vi "Main.vi"(11 "Module Admin":refnum<class "Delacor_lib_QMH_Module Admin.lvclass">) -> ()   [LabVIEW 2024, in "Logger.lvlib"]
doc: "This template is based off of the Queued Message Handler design pattern and the Queued Message Handler project template that ships with LabVIEW.\n\nThe main difference is that the queue is private to this module and communication between modules is performed via Broadcast and Request events.\n\nRequest events are wrapped in public API methods and are handled in the Event Handling Loop (EHL) of this VI. Any module can register for Broadcast events sent by this module. The EHL generates messages based on user interface actions.\n\nThe Message Handling Loop (MHL) processes messages generated by the EHL, or by other messages. The messages are string values, so new messages can be added easily to the Message Cases case structure in the MHL. Each message cluster can also provide an optional value for Message Data, which is a variant that can be converted to whatever message-specific data is required.\n_____\nBased on DQMH Project Template 7.0.0.1280."
uses:
  Logger.lvlib
  <vilib>/Delacor/Delacor QMH/Libraries/Module Admin_class/Delacor_lib_QMH_Module Admin.lvclass
  Module Data--cluster.ctl
  <vilib>/Delacor/Delacor QMH/Libraries/Message Queue_class/Delacor_lib_QMH_Message Queue.lvclass/Delacor_lib_QMH_Message Queue.ctl
  Stop Argument--cluster.ctl
  <vilib>/Delacor/Delacor QMH/Libraries/Module Admin_class/Delacor_lib_QMH_Module Admin.lvclass/Delacor_lib_QMH_Module Admin.ctl
  <vilib>/Utility/miscctls.llb/LVPointTypeDef.ctl
  <vilib>/Delacor/Delacor QMH/Libraries/Message Queue_class/Delacor_lib_QMH_Enqueue Message (Single).vi
  <vilib>/Delacor/Delacor QMH/Libraries/Module Admin_class/Delacor_lib_QMH_Get External Launch.vi
  <vilib>/Delacor/Delacor QMH/Libraries/Message Queue_class/Delacor_lib_QMH_Message Queue.lvclass
panel:
  out "error out":errorcluster
  out "Status":string
  in  "Simulate MHL Error":bool
  in  "Simulate EHL Error":bool
  # "This template is for the DQMH framework. See the block diagram for more information on how to use this template."
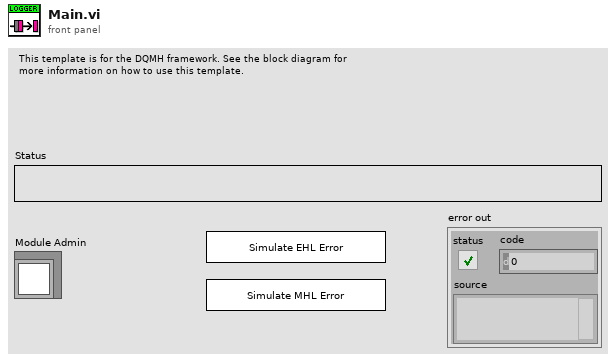
[diagram p1: front panel]
types:
  T1 = typedef "Logger.lvlib/Request Events--cluster.ctl" = cluster{"Stop Module":refnum<user-event>, "Show Panel":refnum<user-event>, "Hide Panel":refnum<user-event>, "Get Module Execution Status":refnum<user-event>, "Show Diagram":refnum<user-event>}
  T2 = typedef "Logger.lvlib/Module Data--cluster.ctl" = cluster{"Status":string}
  T3 = enum32{"invalid lock state", "Not Locked", "Locked (No Password)", "Password-protected"}
  T4 = typedef "Logger.lvlib/Stop Argument--cluster.ctl" = cluster{"Origin":string, "Exit via Stop Module Req?":bool, "Wait for Module to stop?":bool}
  T5 = typedef "LVPointTypeDef.ctl" = cluster{"Horizontal":i16, "Vertical":i16}
  T6 = enum32{"Invalid", "Standard", "Closed", "Hidden", "Minimized", "Maximized"}
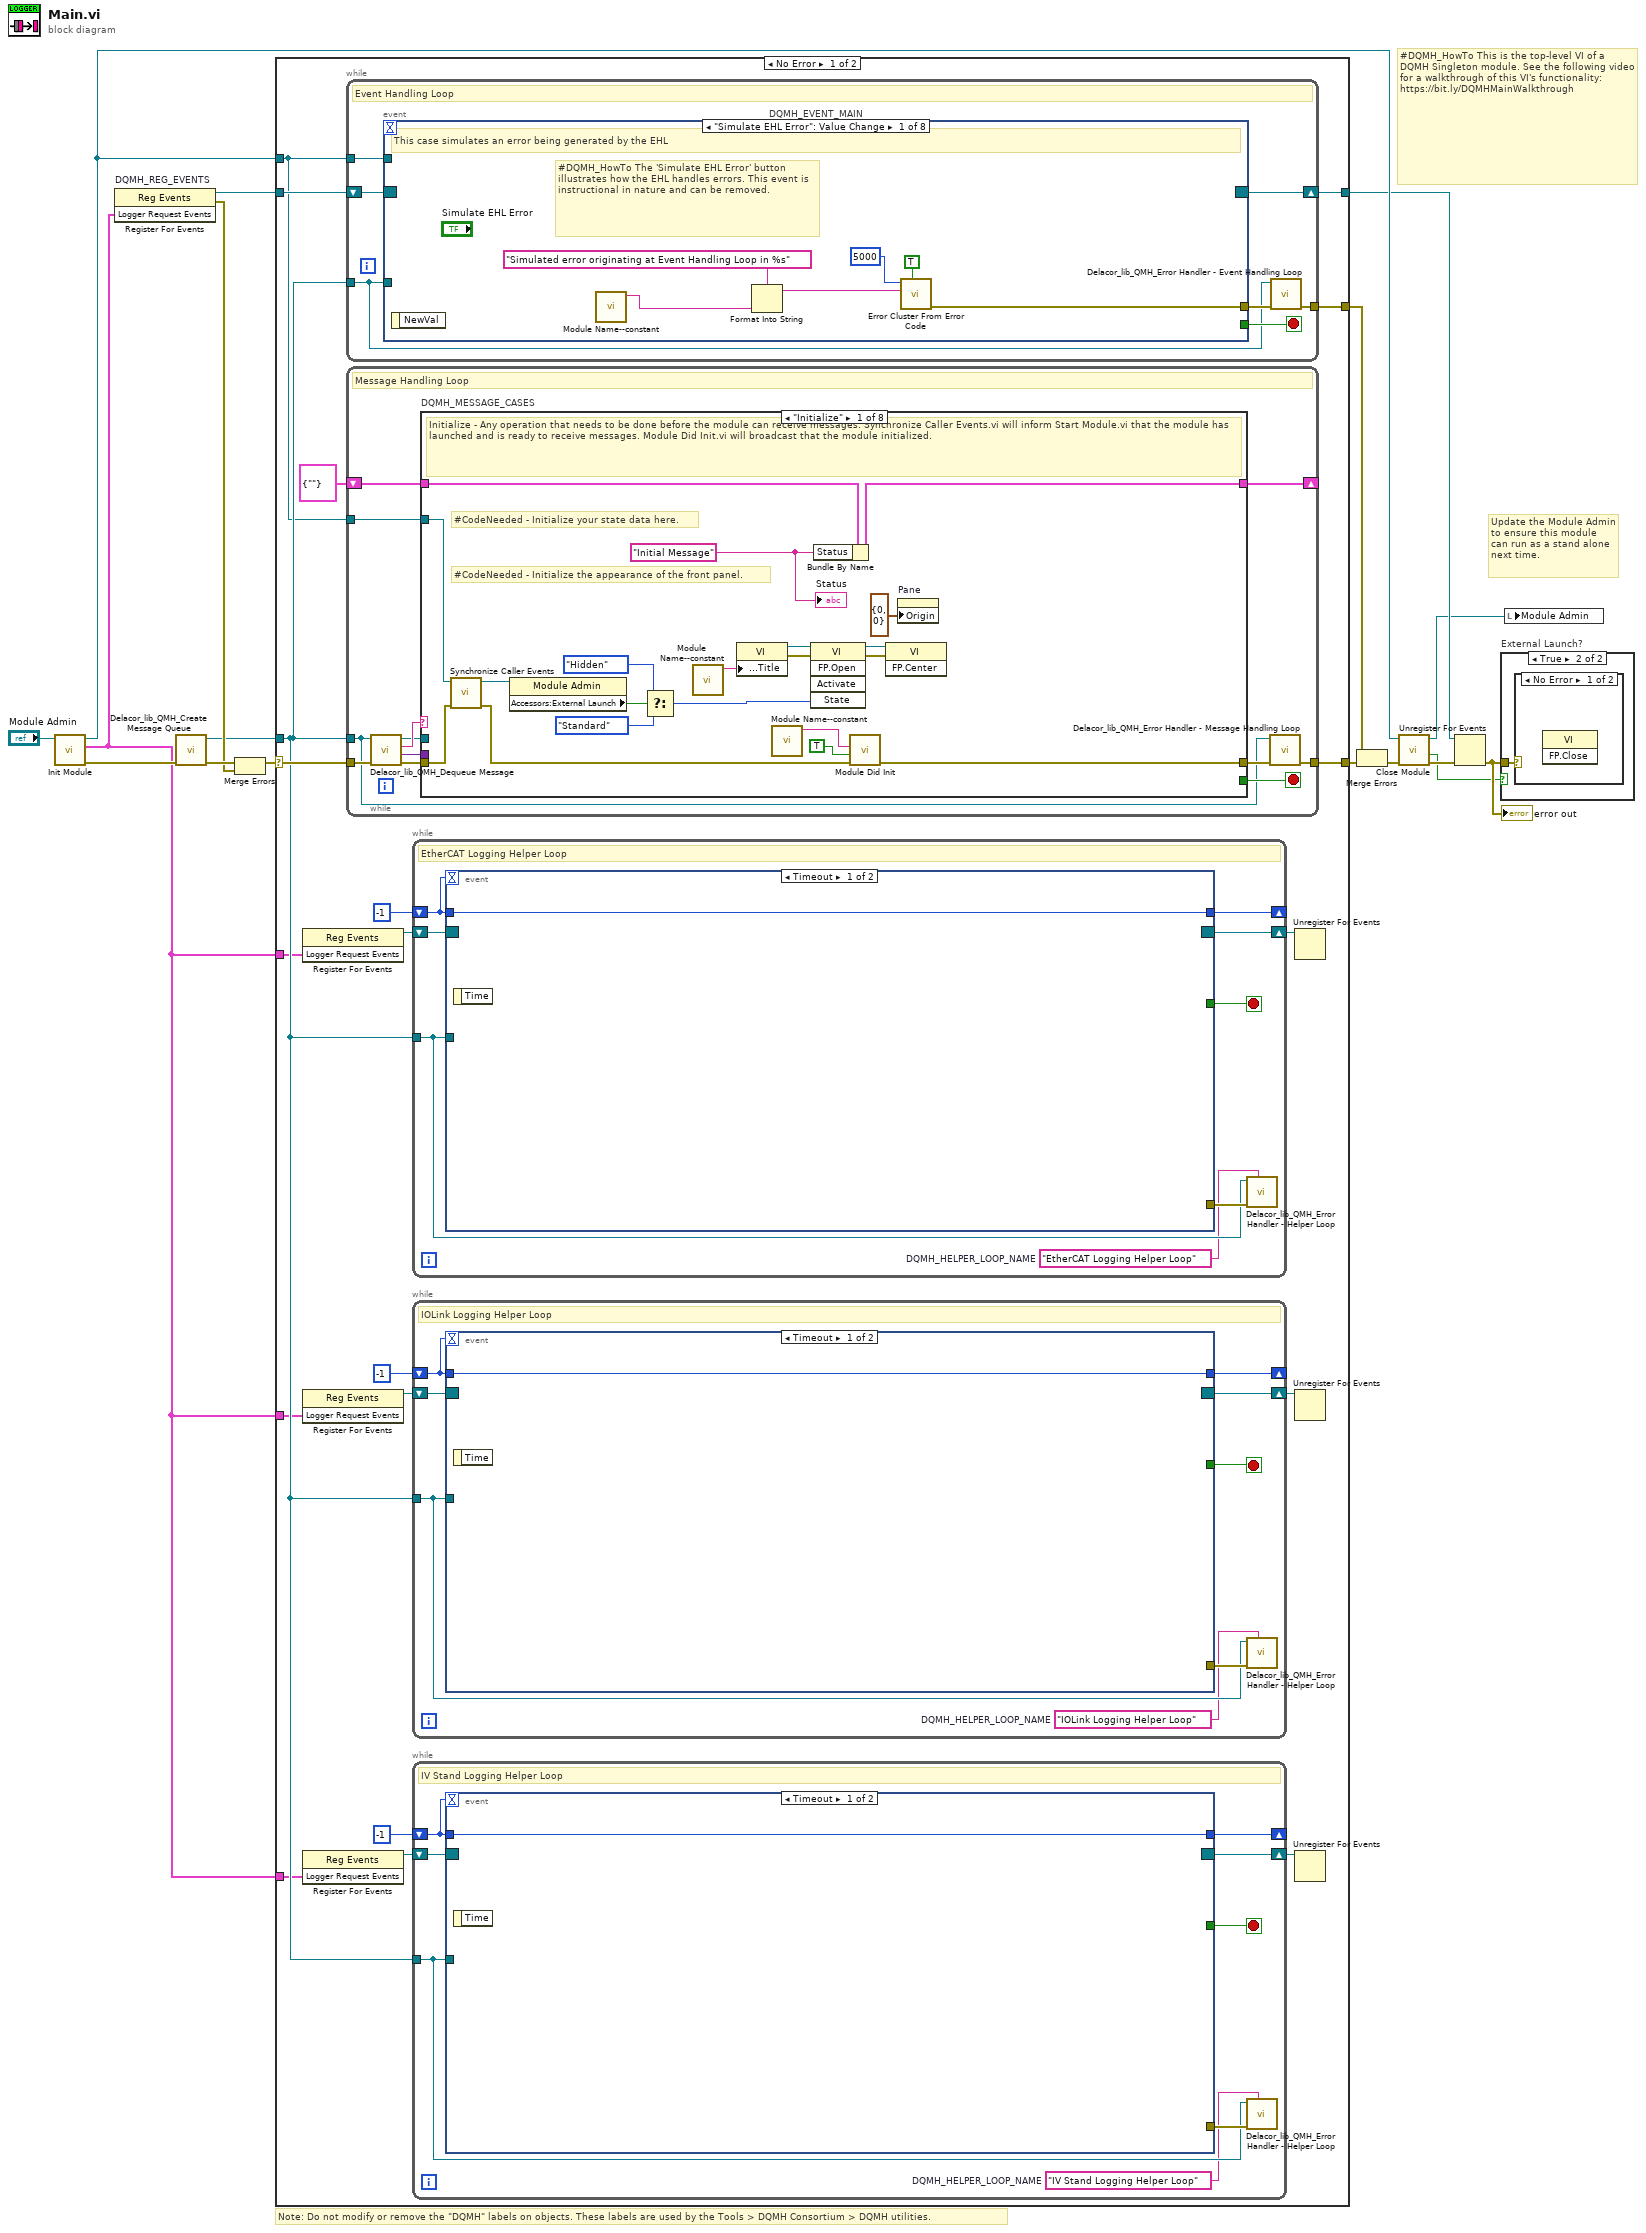
[diagram p0: block diagram]
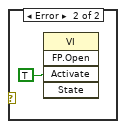
[diagram p3: hidden frame]
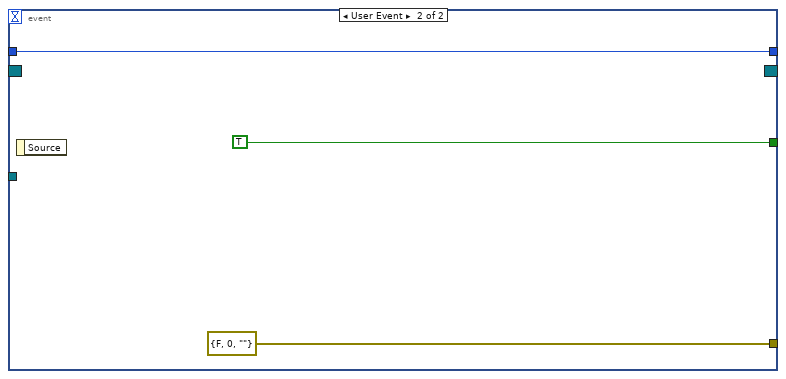
[diagram p4: hidden frame]
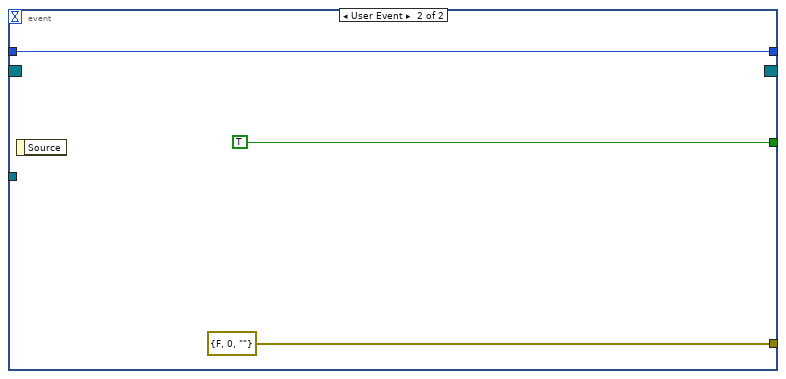
[diagram p5: hidden frame]
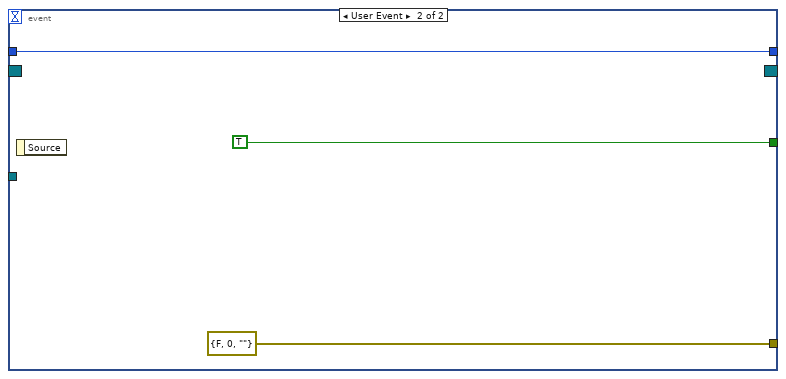
[diagram p6: hidden frame]
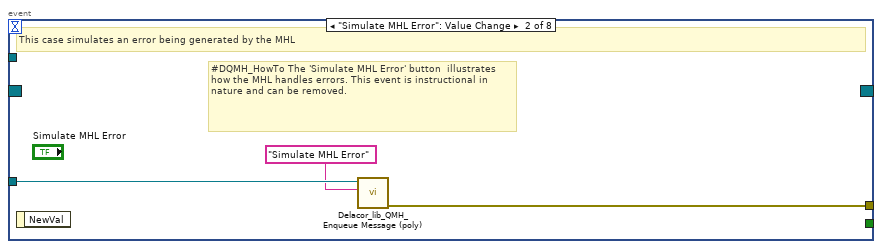
[diagram p7: hidden frame]
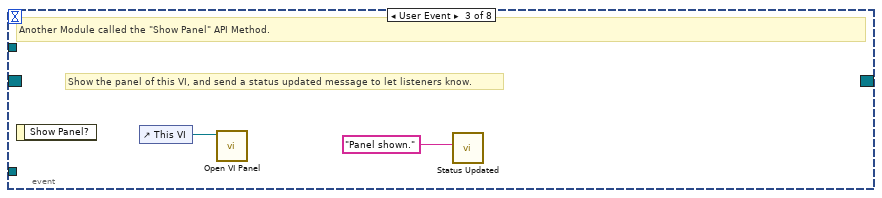
[diagram p8: hidden frame]
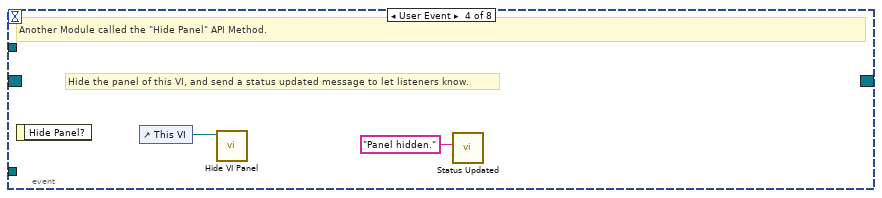
[diagram p9: hidden frame]
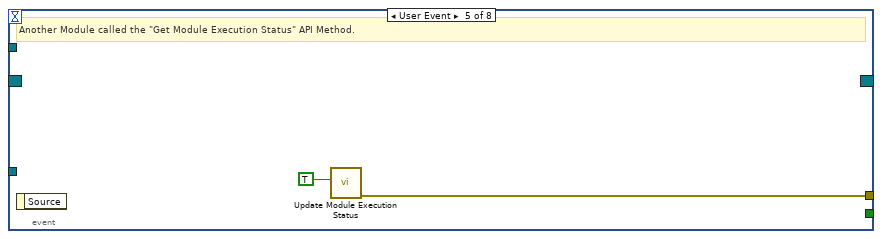
[diagram p10: hidden frame]
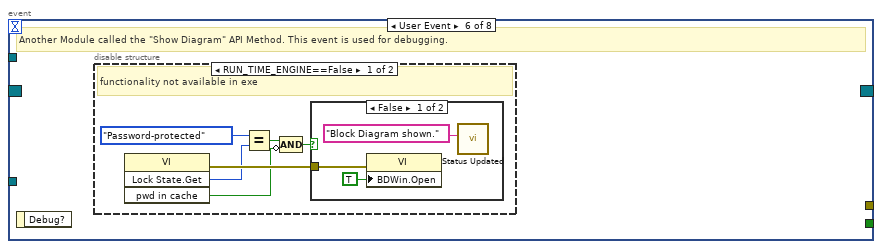
[diagram p11: hidden frame]
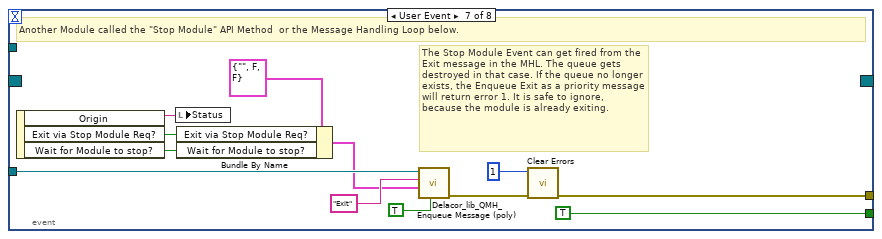
[diagram p14: hidden frame]
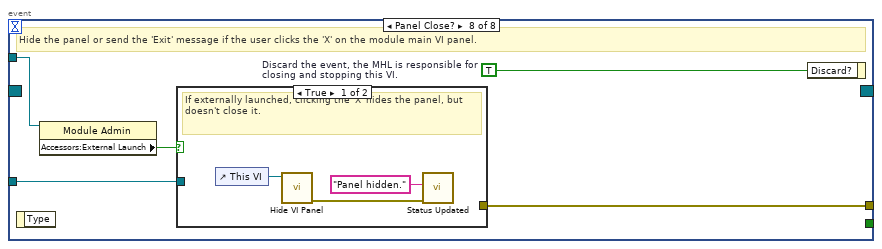
[diagram p15: hidden frame]
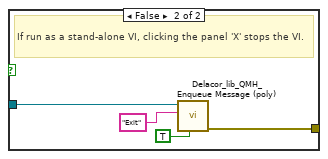
[diagram p16: hidden frame]
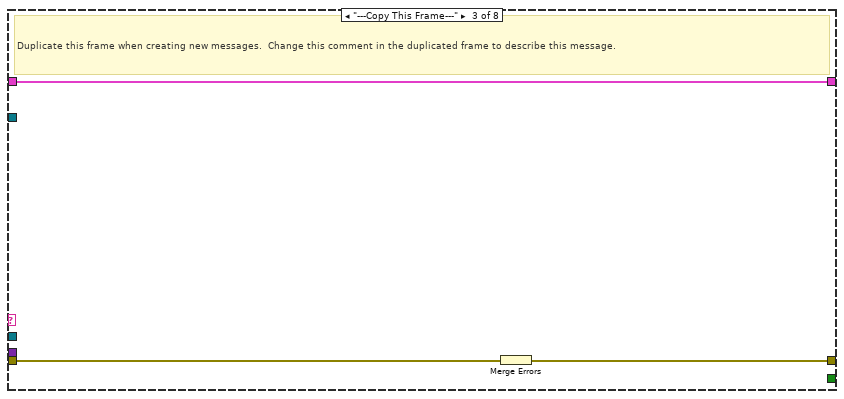
[diagram p18: hidden frame]
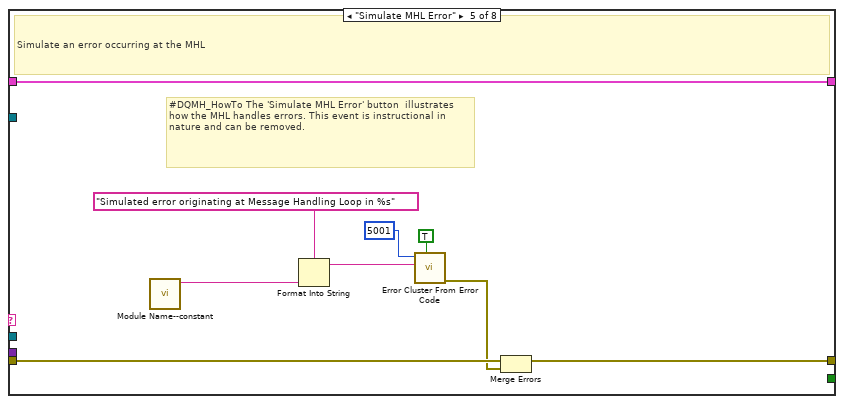
[diagram p20: hidden frame]
diagram:
  # "#DQMH_HowTo This is the top-level VI of a DQMH Singleton module. See the following video for a walkthrough of this VI's functionality: https://bit.ly/DQMHMainWalkthrough"
  # "Note: Do not modify or remove the \"DQMH\" labels on objects. These labels are used by the Tools > DQMH Consortium > DQMH utilities."
  # "Update the Module Admin to ensure this module can run as a stand alone next time."
  n1 = call "Init Module.vi"("Singleton Module Admin in"="Module Admin") -> ("error out"=w16:errorcluster, "Logger Request Events"=w1:T1, "Singleton Module Admin out"=w8:refnum<class "Delacor_lib_QMH_Module Admin.lvclass">)  [unwired: 8 in]
  n2 = register-events "DQMH_REG_EVENTS"(w1) -> (reference out=w6:refnum<event-registration>, error out=w9:errorcluster)  [unwired: 2 in]
  n3 = call <vilib>:"Delacor_lib_QMH_Create Message Queue.vi"("error in"=w16) -> ("error out"=w11:errorcluster, "Message Queue"=w5:refnum<class "Delacor_lib_QMH_Message Queue.lvclass">)  [unwired: 9 in]
  n4 = Merge Errors(w11, w9) -> (w10:errorcluster)
  n5 = case shown="No Error" w10 {
    selector: w10 -> [w35 w226]
    tunnel: [w37 w225] -> w17
    tunnel: [w34 w224] -> w7
    tunnel: w6 -> [w32 w224]
    tunnel: w5 -> [w31 w219]
    tunnel: [w36 _] -> w14
    tunnel: w8 -> [w30 w220]
    tunnel: w1 -> [w29 _]
    tunnel: w1 -> [w25 _]
    tunnel: w1 -> [w21 _]
    frame No Error {
      n6 = register-events ("DQMH_HELPER_REGFOREVENTS")(w29) -> (reference out=w27:refnum<event-registration>)  [unwired: 2 in, 1 out]
      n7 = register-events ("DQMH_HELPER_REGFOREVENTS")(w25) -> (reference out=w23:refnum<event-registration>)  [unwired: 2 in, 1 out]
      n8 = register-events ("DQMH_HELPER_REGFOREVENTS")(w21) -> (reference out=w19:refnum<event-registration>)  [unwired: 2 in, 1 out]
      n9 = while {
        tunnel: w31 -> [w74]
        shift-right: [w77] -> w34
        shift-left: w32 -> [w78]
        tunnel: [w79] -> w36
        tunnel: w30 -> [w75]
        stop <- w76 stop-if-true
        # "Event Handling Loop"
        n10 = event "DQMH_EVENT_MAIN" shown="[0] \"Simulate EHL Error\": Value Change" {
          selector: w78 -> [_ _ _ _ _ _ _ _]
          dyn-events: [_ _ _ _ _ _ _ _] -> w77
          timeout: _ -> [_ _ _ _ _ _ _ _]
          tunnel: [_ _ _ _ _ _ TRUE ("Discard?") _] -> w76
          tunnel: w74 -> [_ w88 _ _ _ _ w112 w119]
          tunnel: [w86 w89 _ _ w95 _ w115 w121] -> w80
          tunnel: w75 -> [_ _ _ _ _ _ _ w118]
          event "Simulate EHL Error": Value Change {
            # "#DQMH_HowTo The 'Simulate EHL Error' button  illustrates how the EHL handles errors. This event is instructional in nature and can be removed."
            # "This case simulates an error being generated by the EHL"
            n11 = event-data() -> ()  [unwired: 1 in, 1 out]
            n12 = call "Module Name--constant.vi"() -> ("Module Name"=w83:string)  [unwired: 11 in]
            n13 = Format Into String(format string="Simulated error originating at Event Handling Loop in %s", w83) -> (resulting string=w84:string)  [unwired: 2 in, 1 out]
            n14 = call <vilib>:"Error Cluster From Error Code.vi"("show call chain? (False)"=TRUE, "error message (\"\")"=w84, "error code (0)"=5000) -> ("error out"=w86:errorcluster)  [unwired: 6 in]
          }
          event "Simulate MHL Error": Value Change {
            # "#DQMH_HowTo The 'Simulate MHL Error' button  illustrates how the MHL handles errors. This event is instructional in nature and can be removed."
            # "This case simulates an error being generated by the MHL"
            n15 = event-data() -> ()  [unwired: 1 in, 1 out]
            n16 = call-poly <vilib>:"Delacor_lib_QMH_Enqueue Message (poly).vi"("Message"="Simulate MHL Error", "Message Queue in"=w88) -> ("error out"=w89:errorcluster)  [unwired: 8 in, 1 out]
          }
          event User Event {
            # "Show the panel of this VI, and send a status updated message to let listeners know."
            # "Another Module called the \"Show Panel\" API Method."
            n17 = event-data() -> ()  [unwired: 1 in, 1 out]
            n18 = control-ref of="This VI"() -> (w91:refnum<vi>)
            n19 = call "Open VI Panel.vi"("VI"=w91) -> ()  [unwired: 10 in, 1 out]
            n20 = call "Status Updated.vi"("Status"="Panel shown." ("format string")) -> ()  [unwired: 10 in, 1 out]
          }
          event User Event {
            # "Hide the panel of this VI, and send a status updated message to let listeners know."
            # "Another Module called the \"Hide Panel\" API Method."
            n21 = event-data() -> ()  [unwired: 1 in, 1 out]
            n22 = control-ref of="This VI"() -> (w93:refnum<vi>)
            n23 = call "Hide VI Panel.vi"("VI"=w93) -> ()  [unwired: 10 in, 1 out]
            n24 = call "Status Updated.vi"("Status"="Panel hidden." ("format string")) -> ()  [unwired: 10 in, 1 out]
          }
          event User Event {
            # "Another Module called the \"Get Module Execution Status\" API Method."
            n25 = event-data() -> ()  [unwired: 1 in, 1 out]
            n26 = call "Update Module Execution Status.vi"("Running?"=TRUE) -> ("error out"=w95:errorcluster)  [unwired: 10 in]
          }
          event User Event {
            # "Another Module called the \"Show Diagram\" API Method. This event is used for debugging."
            n27 = event-data() -> ()  [unwired: 1 in, 1 out]
            n28 = disable-structure shown="RUN_TIME_ENGINE==False" {
              frame condition #0 (active) {
                # "functionality not available in exe"
                n29 = invoke class="VI" method="Lock State.Get"() -> (error out=w101:errorcluster, "Get Lock State"=w100:T3, "pwd in cache"=w97:bool)  [unwired: 4 in, 1 out]
                n30 = Equal?(x=T3."Password-protected", y=w100) -> (x = y?=w98:bool)
                n31 = Compound Arithmetic op=AND(w98, invert w97) -> (w96:bool)
                n32 = case shown="False" w96 {
                  tunnel: w101 -> [w104 _]
                  frame False {
                    n33 = property class="VI"(error in=w104, "BDWin.Open"=TRUE ("Block Diagram Window:Open")) -> ()  [unwired: 1 in, 2 out]
                    n34 = call "Status Updated.vi"("Status"="Block Diagram shown." ("format string")) -> ()  [unwired: 10 in, 1 out]
                  }
                  frame True {
                    # "Password-protected VI, and the password is not in the cache. Do not show the diagram."
                  }
                }
              }
              frame condition #1 {
              }
            }
          }
          event User Event {
            # "The Stop Module Event can get fired from the Exit message in the MHL. The queue gets destroyed in that case. If the queue no longer exists, the Enqueue Exit as a priority message will return error 1. It is safe to ignore, because the module is already exiting."
            # "Another Module called the \"Stop Module\" API Method  or the Message Handling Loop below."
            n35 = event-data() -> ("Origin"=w111:string, "Exit via Stop Module Req?"=w107:bool, "Wait for Module to stop?"=w106:bool)  [unwired: 1 in]
            n36 = local write "Status"(w111) -> ()
            n37 = Bundle By Name(cluster=T4 {"Origin"="", "Exit via Stop Module Req?"=FALSE, "Wait for Module to stop?"=FALSE} ("Stop Argument"), "Exit via Stop Module Req?"=w107, "Wait for Module to stop?"=w106) -> (w105:T4)
            n38 = call-poly <vilib>:"Delacor_lib_QMH_Enqueue Message (poly).vi"("Priority Message? (F)"=TRUE, "Message Data"=w105, "Message"="Exit", "Message Queue in"=w112) -> ("error out"=w116:errorcluster)  [unwired: 6 in, 1 out]
            n39 = call <vilib>:"Clear Errors.vi"("error in (no error)"=w116, "specific error code to clear (0: all)"=1) -> ("error out"=w115:errorcluster)  [unwired: 4 in, 1 out]
          }
          event Panel Close? {
            w120 = TRUE  # Discard the event, the MHL is responsible for closing and stopping this VI.
            # "Hide the panel or send the 'Exit' message if the user clicks the 'X' on the module main VI panel."
            n40 = event-data() -> ()  [unwired: 1 in, 1 out]
            n41 = property class="Module Admin"(reference=w118) -> ("Accessors:External Launch"=w117:bool)  [unwired: 1 in, 2 out]
            n42 = case shown="True" w117 {
              tunnel: w119 -> [_ w127]
              tunnel: [_ w128] -> w121
              frame True {
                # "If externally launched, clicking the 'X' hides the panel, but doesn't close it."
                n43 = control-ref of="This VI"() -> (w124:refnum<vi>)
                n44 = call "Hide VI Panel.vi"("VI"=w124) -> ("error out"=w122:errorcluster)  [unwired: 10 in]
                n45 = call "Status Updated.vi"("error in"=w122, "Status"="Panel hidden." ("format string")) -> ()  [unwired: 9 in, 1 out]
              }
              frame False {
                # "If run as a stand-alone VI, clicking the panel 'X' stops the VI."
                n46 = call-poly <vilib>:"Delacor_lib_QMH_Enqueue Message (poly).vi"("Priority Message? (F)"=TRUE, "Message"="Exit", "Message Queue in"=w127) -> ("error out"=w128:errorcluster)  [unwired: 7 in, 1 out]
              }
            }
            n47 = event-data("Discard?"=w120) -> ()  [unwired: 1 in, 1 out]
          }
        }
        n48 = call-dynamic "Delacor_lib_QMH_Error Handler - Event Handling Loop.vi"("error in"=w80, "Message Queue in"=w74) -> ("dup error in"=w79:errorcluster)  [unwired: 8 in, 1 out]
      }
      n49 = while {
        tunnel: w31 -> [w129]
        shift-right: [w135] -> _
        shift-left: T2 {"Status"=""} ("Data Cluster") -> [w136]
        tunnel: w35 -> [w139]
        tunnel: [w137] -> w37
        tunnel: w30 -> [w130]
        stop <- w134 stop-if-true
        # "Message Handling Loop"
        n50 = call-dynamic "Delacor_lib_QMH_Dequeue Message.vi"("error in"=w139, "Message Queue in"=w129) -> ("error out"=w138:errorcluster, "Message Data"=w132:variant, "Message"=w133:string, "Message Queue out"=w131:refnum<class "Delacor_lib_QMH_Message Queue.lvclass">)  [unwired: 6 in]
        n51 = case "DQMH_MESSAGE_CASES" shown="\"Initialize\"" w133 {
          selector: w133 -> [_ _ _ _ _ _ _ w214]
          tunnel: w131 -> [_ _ _ _ _ w180 w202 _]
          tunnel: w138 -> [w158 w162 w165 w167 w176 w187 w208 w217]
          tunnel: [w156 w162 w164 w167 w175 w183 w203 w218] -> w140
          tunnel: w136 -> [w147 w161 w163 w166 w173 w182 w201 w215]
          tunnel: [w146 w161 w163 w166 w173 w182 w201 w215] -> w135
          tunnel: [_ _ _ _ _ _ w200 _] -> w134
          tunnel: w132 -> [_ _ _ _ _ w181 w199 _]
          tunnel: w130 -> [w148 _ _ _ _ w179 w194 _]
          frame "Initialize" {
            w142 = "Initial Message" ("Initial Message")
            # "#CodeNeeded - Initialize the appearance of the front panel."
            # "#CodeNeeded - Initialize your state data here."
            # "Initialize - Any operation that needs to be done before the module can receive messages. Synchronize Caller Events.vi will inform Start Module.vi that the module has launched and is ready to receive messages. Module Did Init.vi will broadcast that the module initialized."
            n52 = call "Synchronize Caller Events.vi"("error in"=w158, "Singleton Module Admin in"=w148) -> ("error out"=w157:errorcluster, "Singleton Module Admin out"=w143:refnum<class "Delacor_lib_QMH_Module Admin.lvclass">)  [unwired: 8 in]
            n53 = property class="Module Admin"(reference=w143) -> ("Accessors:External Launch"=w152:bool)  [unwired: 1 in, 2 out]
            n54 = Select(t=T6."Hidden" ("State"), s=w152, f=T6."Standard" ("State")) -> (s? t:f=w149:T6)
            n55 = call "Module Name--constant.vi"() -> ("Module Name"=w155:string)  [unwired: 11 in]
            n56 = property class="VI"("Front Panel.Title"=w155) -> (reference out=w154:refnum<vi>, error out=w160:errorcluster)  [unwired: 2 in]
            n57 = call "Module Name--constant.vi"() -> ("Module Name"=w144:string)  [unwired: 11 in]
            n58 = invoke class="VI" method="FP.Open"(reference=w154, error in=w160, "State"=w149) -> (reference out=w153:refnum<vi>, error out=w159:errorcluster)  [unwired: 2 in, 3 out]
            n59 = Bundle By Name(cluster=w147, "Status"=w142) -> (w146:T2)
            n60 = call "Module Did Init.vi"("error in"=w157, "Initialized?"=TRUE, "Origin"=w144) -> ("error out"=w156:errorcluster)  [unwired: 8 in]
            n61 = invoke class="VI" method="FP.Center"(reference=w153, error in=w159) -> ()  [unwired: 1 in, 3 out]
            n62 = property on="Pane" class="Pane"("Origin"=T5 {"Horizontal"=0, "Vertical"=0}) -> ()  [unwired: 2 in, 2 out]
            "Status" <- w142
          }
          frame "---Module Specific---" {
            # "Separator -- The following cases handle messages specific to this Module."
          }
          frame "---Copy This Frame---" {
            # "Duplicate this frame when creating new messages.  Change this comment in the duplicated frame to describe this message."
            n63 = Merge Errors(w165) -> (w164:errorcluster)
          }
          frame "---Exit and Error Handling---" {
            # "Separator - The following cases handle errors and exit messages."
          }
          frame "Simulate MHL Error" {
            # "#DQMH_HowTo The 'Simulate MHL Error' button  illustrates how the MHL handles errors. This event is instructional in nature and can be removed."
            # "Simulate an error occurring at the MHL"
            n64 = call "Module Name--constant.vi"() -> ("Module Name"=w169:string)  [unwired: 11 in]
            n65 = Format Into String(format string="Simulated error originating at Message Handling Loop in %s", w169) -> (resulting string=w170:string)  [unwired: 2 in, 1 out]
            n66 = call <vilib>:"Error Cluster From Error Code.vi"("show call chain? (False)"=TRUE, "error message (\"\")"=w170, "error code (0)"=5001) -> ("error out"=w174:errorcluster)  [unwired: 6 in]
            n67 = Merge Errors(w176, w174) -> (w175:errorcluster)
          }
          frame "Error" {
            # "#CodeRecommended - If the module is running in standalone mode (External Launch = FALSE), this code will pop up an error dialog and call the 'Exit' message if an error occurs. Add more fine-grained error management here."
            # "Error - Check the error message data and respond accordingly. This message is sent by the \"Error Handler\" VIs at the end of each loop in this application."
            n68 = property class="Module Admin"(reference=w179) -> ("Accessors:External Launch"=w178:bool)  [unwired: 1 in, 2 out]
            n69 = Variant To Data(error in=w187, type=errorcluster {"status"=FALSE, "code"=0, "source"=""} ("error constant"), Variant=w181) -> (data=w177:errorcluster, error out=w185:errorcluster)
            n70 = local write "error out"(w177) -> ()
            n71 = call "Error Reported.vi"("Error"=w177) -> ()  [unwired: 10 in, 1 out]
            n72 = case shown="False" w178 {
              tunnel: [w192 _] -> w184
              tunnel: w180 -> [w190 _]
              tunnel: w177 -> [w191 _]
              frame False {
                n73 = disable-structure shown="Default" {
                  disable-tunnel: w191 -> [w193 _]
                  frame condition #0 (active) {
                    # "If the module is running standalone, then pop up an error dialog and call the \"Exit\" message."
                    n74 = call <vilib>:"Simple Error Handler.vi"("error in (no error)"=w193) -> ()  [unwired: 4 in, 5 out]
                  }
                  frame condition #1 {
                    # "To prevent the Simple Error Handler VI from being loaded (e.g. when deploying to a Real-Time target), add the Conditional Disable Symbol \"DQMH_Disable_SEH\" to your project and set it to TRUE."
                  }
                }
                n75 = call-poly <vilib>:"Delacor_lib_QMH_Enqueue Message (poly).vi"("Priority Message? (F)"=TRUE, "Message"="Exit", "Message Queue in"=w190) -> ("error out"=w192:errorcluster)  [unwired: 7 in, 1 out]
              }
              frame True {
                # "If the module was launched externally, calling the Error Reported broadcast VI is the only action performed by the \"Error\" message. The module's caller can then process the error appropriately."
              }
            }
            n76 = Merge Errors(w185, w184) -> (w183:errorcluster)
          }
          frame "Exit" {
            w198 = 91  # 91: not all Exit messages will have an argument
            w200 = TRUE  # Stop the VI
            # "Release the message queue reference"
            # "#CodeNeeded - Add any required cleanup code here."
            # "Exit - Exit the application."
            n77 = Variant To Data(error in=w208, type=T4 {"Origin"="", "Exit via Stop Module Req?"=FALSE, "Wait for Module to stop?"=FALSE} ("Stop Argument"), Variant=w199) -> (data=w196:T4, error out=w205:errorcluster)
            n78 = call <vilib>:"Clear Errors.vi"("error in (no error)"=w205, "specific error code to clear (0: all)"=w198) -> ("error out"=w207:errorcluster)  [unwired: 4 in, 1 out]
            n79 = control-ref of="This VI"() -> (w195:refnum<vi>)
            n80 = call-dynamic "Delacor_lib_QMH_Release Message Queue.vi"("error in"=w207, "Message Queue"=w202) -> ("error out"=w206:errorcluster)  [unwired: 9 in]
            n81 = call "Handle Exit.vi"("Stop Argument"=w196, "Admin in"=w194, "VI reference"=w195) -> ("error out"=w204:errorcluster)  [unwired: 7 in, 1 out]
            n82 = Merge Errors(w206, w204) -> (w203:errorcluster)
            n83 = call "Error Reported.vi"("Error"=w203) -> ()  [unwired: 10 in, 1 out]
          }
          frame Default {
            # "'Default' case only runs if there is a message that isn't defined in any of the other cases.  Output a programming error."
            n84 = call "Module Name--constant.vi"() -> ("Module Name"=w213:string)  [unwired: 11 in]
            n85 = Format Into String(format string="The invalid message string \"%s\" was received in the Message Handling Loop for module \"%s\".", w214, w213) -> (resulting string=w209:string)  [unwired: 2 in, 1 out]
            n86 = call <vilib>:"Error Cluster From Error Code.vi"("show call chain? (False)"=TRUE, "error message (\"\")"=w209, "error code (0)"=1) -> ("error out"=w216:errorcluster)  [unwired: 6 in]
            n87 = Merge Errors(w217, w216) -> (w218:errorcluster)
          }
        }
        n88 = call-dynamic "Delacor_lib_QMH_Error Handler - Message Handling Loop.vi"("error in"=w140, "Message Queue in"=w129) -> ("dup error in"=w137:errorcluster)  [unwired: 8 in, 1 out]
      }
      n89 = while "DQMH_HELPER_LOOP" {
        shift-right: [w69] -> _
        shift-left: -1 -> [w68]
        shift-right: [w66] -> w28
        shift-left: w27 -> [w67]
        tunnel: w31 -> [w63]
        stop <- w65 stop-if-true
        w62 = "EtherCAT Logging Helper Loop"  # DQMH_HELPER_LOOP_NAME
        # "EtherCAT Logging Helper Loop"
        n90 = event "DQMH_HELPER_EVENT_STRUCTURE" shown="[0] Timeout" {
          selector: w67 -> [_ _]
          dyn-events: [_ _] -> w66
          timeout: w68 -> [_ _]
          tunnel: w68 -> [w70 w73]
          tunnel: [w70 w73] -> w69
          tunnel: [_ TRUE] -> w65
          tunnel: [_ errorcluster {"status"=FALSE, "code"=0, "source"=""} ("error constant")] -> w64
          tunnel: w63 -> [_ _]
          event Timeout {
            n91 = event-data() -> ()  [unwired: 1 in, 1 out]
          }
          event User Event {
            n92 = event-data() -> ()  [unwired: 1 in, 1 out]
          }
        }
        n93 = call-dynamic "Delacor_lib_QMH_Error Handler - Helper Loop.vi"("Error Debug"=w62, "error in"=w64, "Message Queue in"=w63) -> ()  [unwired: 7 in, 2 out]
      }
      n94 = while "DQMH_HELPER_LOOP" {
        shift-right: [w57] -> _
        shift-left: -1 -> [w56]
        shift-right: [w54] -> w24
        shift-left: w23 -> [w55]
        tunnel: w31 -> [w51]
        stop <- w53 stop-if-true
        w50 = "IOLink Logging Helper Loop"  # DQMH_HELPER_LOOP_NAME
        # "IOLink Logging Helper Loop"
        n95 = event "DQMH_HELPER_EVENT_STRUCTURE" shown="[0] Timeout" {
          selector: w55 -> [_ _]
          dyn-events: [_ _] -> w54
          timeout: w56 -> [_ _]
          tunnel: w56 -> [w58 w61]
          tunnel: [w58 w61] -> w57
          tunnel: [_ TRUE] -> w53
          tunnel: [_ errorcluster {"status"=FALSE, "code"=0, "source"=""} ("error constant")] -> w52
          tunnel: w51 -> [_ _]
          event Timeout {
            n96 = event-data() -> ()  [unwired: 1 in, 1 out]
          }
          event User Event {
            n97 = event-data() -> ()  [unwired: 1 in, 1 out]
          }
        }
        n98 = call-dynamic "Delacor_lib_QMH_Error Handler - Helper Loop.vi"("Error Debug"=w50, "error in"=w52, "Message Queue in"=w51) -> ()  [unwired: 7 in, 2 out]
      }
      n99 = while "DQMH_HELPER_LOOP" {
        shift-right: [w45] -> _
        shift-left: -1 -> [w44]
        shift-right: [w42] -> w20
        shift-left: w19 -> [w43]
        tunnel: w31 -> [w39]
        stop <- w41 stop-if-true
        w38 = "IV Stand Logging Helper Loop"  # DQMH_HELPER_LOOP_NAME
        # "IV Stand Logging Helper Loop"
        n100 = event "DQMH_HELPER_EVENT_STRUCTURE" shown="[0] Timeout" {
          selector: w43 -> [_ _]
          dyn-events: [_ _] -> w42
          timeout: w44 -> [_ _]
          tunnel: w44 -> [w46 w49]
          tunnel: [w46 w49] -> w45
          tunnel: [_ TRUE] -> w41
          tunnel: [_ errorcluster {"status"=FALSE, "code"=0, "source"=""} ("error constant")] -> w40
          tunnel: w39 -> [_ _]
          event Timeout {
            n101 = event-data() -> ()  [unwired: 1 in, 1 out]
          }
          event User Event {
            n102 = event-data() -> ()  [unwired: 1 in, 1 out]
          }
        }
        n103 = call-dynamic "Delacor_lib_QMH_Error Handler - Helper Loop.vi"("Error Debug"=w38, "error in"=w40, "Message Queue in"=w39) -> ()  [unwired: 7 in, 2 out]
      }
      n104 = Unregister For Events(event registration refnum=w28) -> ()  [unwired: 1 in, 1 out]
      n105 = Unregister For Events(event registration refnum=w24) -> ()  [unwired: 1 in, 1 out]
      n106 = Unregister For Events(event registration refnum=w20) -> ()  [unwired: 1 in, 1 out]
    }
    frame Error {
      # "Synchronize Caller Events.vi will inform Start Module.vi that the module has launched and will let the code calling Start Module.vi register for broadcasts and would permit the caller receive the broadcast that an error occurred at launch time."
      n107 = call-dynamic "Delacor_lib_QMH_Release Message Queue.vi"("error in"=w226, "Message Queue"=w219) -> ("error out"=w225:errorcluster)  [unwired: 9 in]
      n108 = call "Synchronize Caller Events.vi"("Singleton Module Admin in"=w220) -> ("error out"=w227:errorcluster)  [unwired: 9 in, 1 out]
      n109 = call "Module Name--constant.vi"() -> ("Module Name"=w223:string)  [unwired: 11 in]
      n110 = Format Into String(format string="An error occurred during initialization. %s is no longer running.", w223) -> (resulting string=w221:string)  [unwired: 2 in, 1 out]
      n111 = Merge Errors(w225, w227) -> (w228:errorcluster)
      n112 = call "Error Reported.vi"("Additional Information"=w221, "Error"=w228) -> ()  [unwired: 9 in, 1 out]
    }
  }
  n113 = Merge Errors(w14, w17) -> (w13:errorcluster)
  n114 = call "Close Module.vi"("error in"=w13, "Module Admin in"=w8) -> ("error out"=w15:errorcluster, "External Launch"=w2:bool, "Module Admin out"=w3:refnum<class "Delacor_lib_QMH_Module Admin.lvclass">)  [unwired: 7 in]
  n115 = Unregister For Events(event registration refnum=w7, error in=w15) -> (error out=w12:errorcluster)
  "error out" <- w12
  n116 = case "External Launch?" shown="True" w2 {
    tunnel: w12 -> [_ w229]
    frame False {
    }
    frame True {
      n117 = case shown="No Error" w229 {
        frame No Error {
          n118 = invoke class="VI" method="FP.Close"() -> ()  [unwired: 3 in, 3 out]
        }
        frame Error {
          n119 = invoke class="VI" method="FP.Open"("Activate"=TRUE ("Activate?")) -> ()  [unwired: 4 in, 5 out]
        }
      }
    }
  }
  n120 = local write "Module Admin"(w3) -> ()
